vi "PT100Read.vi"(11 "TI XX":dbl) -> (3 "temp":dbl)   [LabVIEW 2020]
doc: "Computes temperature equivalent from voltage read at the output of the conditioning circuit for the PT100."
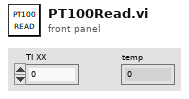
[diagram p1: front panel]
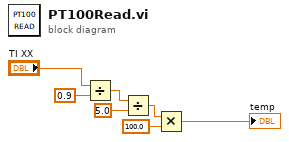
[diagram p0: block diagram]
diagram:
  n1 = Divide(x="TI XX", y=0.9) -> (x/y=w3:dbl)
  n2 = Divide(x=w3, y=5.0) -> (x/y=w5:dbl)
  n3 = Multiply(x=w5, y=100.0) -> (x*y=→"temp":dbl)
